vi "AutoEncoder_demo.vi"() -> ()   [LabVIEW 2014]
uses:
  <vilib>/Analysis/baseanly.llb/Vector x A.vi
  <vilib>/Analysis/baseanly.llb/A x Vector.vi
  <vilib>/Analysis/NI_AALBase.lvlib
panel:
  out "XY Graph":cluster{"Array":i32[], dbl[]}(graph)={"Array"=[0, 1, 2, 3, 4, 5, 6, 7, 8, 9, 10, 11, 12, 13, 14, 15, 16, 17, 18, 19, 20, 21, 22, 23, 24, 25, 26, 27, 28, 29, 30, 31, 32, 33, 34, 35, 36, 37, 38, 39, 40, 41, 42, 43, 44, 45, 46, 47, 48, 49, 50, 51, 52, 53, 54, 55, 56, 57, 58, 59, 60, 61, 62, 63, 64, 65, 66, 67, 68, 69, 70, 71, 72, 73, 74, 75, 76, 77, 78, 79, 80, 81, 82, 83, 84, 85, 86, 87, 88, 89, 90, 91, 92, 93, 94, 95, 96, 97, 98, 99, 100, 101, 102, 103, 104, 105, 106, 107, 108, 109, 110, 111, 112, 113, 114, 115, 116, 117, 118, 119, 120, 121, 122, 123, 124, 125, 126, 127, 128, 129, 130, 131, 132, 133, 134, 135, 136, 137, 138, 139, 140, 141, 142, 143, 144, 145, 146, 147, 148, 149, 150], [4.302449553595711, 4.048227484741284, 4.531011299054813, 7.377745697197833, 5.077085434012255, 3.4640879938686306, 2.3579555059462405, 1.6031005412667185, 1.0891350906968578, 0.7396289977203222, 0.5021401051785775, 0.340844705599286, 0.2313319633254815, 0.15699277846584656, 0.10653694142375755, 0.07229445990475002, 0.04905680313771316, 0.03328790003409601, 0.02258753540240982, 0.01532668338521762, 0.010399812316621135, 0.007056697956674369, 0.004788249443257091, 0.003249013786339784, 0.0022045813097912245, 0.0014958933253162794, 0.0010150213329413618, 0.0006887313161076235, 0.0004673310693692157, 0.0003171025081088373, 0.0002151666308504492, 0.00014599917380717274, 9.90663411896271e-05, 6.722055641586043e-05, 4.561191871794354e-05, 3.094958594365995e-05, 2.1000595504256945e-05, 1.4249795896008899e-05, 9.669097646393528e-06, 6.560901500715122e-06, 4.451858575365319e-06, 3.0207826056200174e-06, 2.049735653954206e-06, 1.3908378815287861e-06, 9.43746682957844e-07, 6.403753963009146e-07, 4.3452434133222085e-07, 2.9484505986245243e-07, 2.0006626981382739e-07, 1.357544787687443e-07, 9.211592856751061e-08, 6.250511769704593e-08, 4.241277514149957e-08, 2.8779157426316175e-08, 1.952808890997346e-08, 1.325078707523578e-08, 8.991329075107176e-09, 6.101075692115192e-09, 4.139893199625439e-09, 2.8091322905979654e-09, 1.9061429298950496e-09, 1.2934183593129547e-09, 8.776533856361072e-10, 5.955344848861016e-10, 4.0410240849601025e-10, 2.742056229699723e-10, 1.86063528240424e-10, 1.262547911345823e-10, 8.567078053512786e-11, 5.813246002910622e-11, 3.9445781999185135e-11, 2.676665895782682e-11, 1.8162552403284542e-11, 1.2324148813570466e-11, 8.362283563934942e-12, 5.67446040597241e-12, 3.8502652326963085e-12, 2.6127838590636877e-12, 1.7730125366726473e-12, 1.2031418508383047e-12, 8.164299826220104e-13, 5.538626219870757e-13, 3.758294302867062e-13, 2.550782897881239e-13, 1.7319293256381905e-13, 1.1743050459643337e-13, 7.965906292895184e-14, 5.4198843464053e-14, 3.6641859303897325e-14, 2.5087294302303138e-14, 1.7116730937182402e-14, 1.1708807263476445e-14, 8.099683797877964e-15, 5.511072057502669e-15, 3.751420436264963e-15, 2.6978647938375716e-15, 1.8569289088252427e-15, 1.59250260620481e-15, 1.1240151438116956e-15, 9.914608633805194e-16, 9.773746735086136e-16, 9.662767911105659e-16, 7.570711667007543e-16, 7.570711667007543e-16, 7.570711667007543e-16, 7.570711667007543e-16, 7.570711667007543e-16, 7.570711667007543e-16, 7.570711667007543e-16, 6.888752704931532e-16, 6.888752704931532e-16, 6.888752704931532e-16, 6.888752704931532e-16, 6.888752704931532e-16, 6.888752704931532e-16, 6.888752704931532e-16, 6.888752704931532e-16, 6.888752704931532e-16, 6.888752704931532e-16, 6.888752704931532e-16, 6.888752704931532e-16, 6.888752704931532e-16, 6.888752704931532e-16, 6.888752704931532e-16, 6.521083742145178e-16, 6.521083742145178e-16, 6.521083742145178e-16, 6.521083742145178e-16, 6.521083742145178e-16, 6.521083742145178e-16, 6.521083742145178e-16, 6.521083742145178e-16, 6.521083742145178e-16, 6.521083742145178e-16, 6.521083742145178e-16, 6.521083742145178e-16, 6.521083742145178e-16, 6.521083742145178e-16, 6.521083742145178e-16, 6.521083742145178e-16, 6.521083742145178e-16, 6.521083742145178e-16, 6.521083742145178e-16, 6.521083742145178e-16, 6.521083742145178e-16, 6.521083742145178e-16, 6.521083742145178e-16, 6.521083742145178e-16, 6.521083742145178e-16, 6.521083742145178e-16, 6.521083742145178e-16]}
  out "Waveform Chart":dbl[](graph)=[4.302449553595711, 4.048227484741284, 4.531011299054813, 7.377745697197833, 5.077085434012255, 3.4640879938686306, 2.3579555059462405, 1.6031005412667185, 1.0891350906968578, 0.7396289977203222, 0.5021401051785775, 0.340844705599286, 0.2313319633254815, 0.15699277846584656, 0.10653694142375755, 0.07229445990475002, 0.04905680313771316, 0.03328790003409601, 0.02258753540240982, 0.01532668338521762, 0.010399812316621135, 0.007056697956674369, 0.004788249443257091, 0.003249013786339784, 0.0022045813097912245, 0.0014958933253162794, 0.0010150213329413618, 0.0006887313161076235, 0.0004673310693692157, 0.0003171025081088373, 0.0002151666308504492, 0.00014599917380717274, 9.90663411896271e-05, 6.722055641586043e-05, 4.561191871794354e-05, 3.094958594365995e-05, 2.1000595504256945e-05, 1.4249795896008899e-05, 9.669097646393528e-06, 6.560901500715122e-06, 4.451858575365319e-06, 3.0207826056200174e-06, 2.049735653954206e-06, 1.3908378815287861e-06, 9.43746682957844e-07, 6.403753963009146e-07, 4.3452434133222085e-07, 2.9484505986245243e-07, 2.0006626981382739e-07, 1.357544787687443e-07, 9.211592856751061e-08, 6.250511769704593e-08, 4.241277514149957e-08, 2.8779157426316175e-08, 1.952808890997346e-08, 1.325078707523578e-08, 8.991329075107176e-09, 6.101075692115192e-09, 4.139893199625439e-09, 2.8091322905979654e-09, 1.9061429298950496e-09, 1.2934183593129547e-09, 8.776533856361072e-10, 5.955344848861016e-10, 4.0410240849601025e-10, 2.742056229699723e-10, 1.86063528240424e-10, 1.262547911345823e-10, 8.567078053512786e-11, 5.813246002910622e-11, 3.9445781999185135e-11, 2.676665895782682e-11, 1.8162552403284542e-11, 1.2324148813570466e-11, 8.362283563934942e-12, 5.67446040597241e-12, 3.8502652326963085e-12, 2.6127838590636877e-12, 1.7730125366726473e-12, 1.2031418508383047e-12, 8.164299826220104e-13, 5.538626219870757e-13, 3.758294302867062e-13, 2.550782897881239e-13, 1.7319293256381905e-13, 1.1743050459643337e-13, 7.965906292895184e-14, 5.4198843464053e-14, 3.6641859303897325e-14, 2.5087294302303138e-14, 1.7116730937182402e-14, 1.1708807263476445e-14, 8.099683797877964e-15, 5.511072057502669e-15, 3.751420436264963e-15, 2.6978647938375716e-15, 1.8569289088252427e-15, 1.59250260620481e-15, 1.1240151438116956e-15, 9.914608633805194e-16, 9.773746735086136e-16, 9.662767911105659e-16, 7.570711667007543e-16, 7.570711667007543e-16, 7.570711667007543e-16, 7.570711667007543e-16, 7.570711667007543e-16, 7.570711667007543e-16, 7.570711667007543e-16, 6.888752704931532e-16, 6.888752704931532e-16, 6.888752704931532e-16, 6.888752704931532e-16, 6.888752704931532e-16, 6.888752704931532e-16, 6.888752704931532e-16, 6.888752704931532e-16, 6.888752704931532e-16, 6.888752704931532e-16, 6.888752704931532e-16, 6.888752704931532e-16, 6.888752704931532e-16, 6.888752704931532e-16, 6.888752704931532e-16, 6.521083742145178e-16, 6.521083742145178e-16, 6.521083742145178e-16, 6.521083742145178e-16, 6.521083742145178e-16, 6.521083742145178e-16, 6.521083742145178e-16, 6.521083742145178e-16, 6.521083742145178e-16, 6.521083742145178e-16, 6.521083742145178e-16, 6.521083742145178e-16, 6.521083742145178e-16, 6.521083742145178e-16, 6.521083742145178e-16, 6.521083742145178e-16, 6.521083742145178e-16, 6.521083742145178e-16, 6.521083742145178e-16, 6.521083742145178e-16, 6.521083742145178e-16, 6.521083742145178e-16, 6.521083742145178e-16, 6.521083742145178e-16, 6.521083742145178e-16, 6.521083742145178e-16, 6.521083742145178e-16]
  out "Total Error":dbl[](array[numeric])=[4.302449553595711, 4.048227484741284, 4.531011299054813, 7.377745697197833, 5.077085434012255, 3.4640879938686306, 2.3579555059462405, 1.6031005412667185, 1.0891350906968578, 0.7396289977203222, 0.5021401051785775, 0.340844705599286, 0.2313319633254815, 0.15699277846584656, 0.10653694142375755, 0.07229445990475002, 0.04905680313771316, 0.03328790003409601, 0.02258753540240982, 0.01532668338521762, 0.010399812316621135, 0.007056697956674369, 0.004788249443257091, 0.003249013786339784, 0.0022045813097912245, 0.0014958933253162794, 0.0010150213329413618, 0.0006887313161076235, 0.0004673310693692157, 0.0003171025081088373, 0.0002151666308504492, 0.00014599917380717274, 9.90663411896271e-05, 6.722055641586043e-05, 4.561191871794354e-05, 3.094958594365995e-05, 2.1000595504256945e-05, 1.4249795896008899e-05, 9.669097646393528e-06, 6.560901500715122e-06, 4.451858575365319e-06, 3.0207826056200174e-06, 2.049735653954206e-06, 1.3908378815287861e-06, 9.43746682957844e-07, 6.403753963009146e-07, 4.3452434133222085e-07, 2.9484505986245243e-07, 2.0006626981382739e-07, 1.357544787687443e-07, 9.211592856751061e-08, 6.250511769704593e-08, 4.241277514149957e-08, 2.8779157426316175e-08, 1.952808890997346e-08, 1.325078707523578e-08, 8.991329075107176e-09, 6.101075692115192e-09, 4.139893199625439e-09, 2.8091322905979654e-09, 1.9061429298950496e-09, 1.2934183593129547e-09, 8.776533856361072e-10, 5.955344848861016e-10, 4.0410240849601025e-10, 2.742056229699723e-10, 1.86063528240424e-10, 1.262547911345823e-10, 8.567078053512786e-11, 5.813246002910622e-11, 3.9445781999185135e-11, 2.676665895782682e-11, 1.8162552403284542e-11, 1.2324148813570466e-11, 8.362283563934942e-12, 5.67446040597241e-12, 3.8502652326963085e-12, 2.6127838590636877e-12, 1.7730125366726473e-12, 1.2031418508383047e-12, 8.164299826220104e-13, 5.538626219870757e-13, 3.758294302867062e-13, 2.550782897881239e-13, 1.7319293256381905e-13, 1.1743050459643337e-13, 7.965906292895184e-14, 5.4198843464053e-14, 3.6641859303897325e-14, 2.5087294302303138e-14, 1.7116730937182402e-14, 1.1708807263476445e-14, 8.099683797877964e-15, 5.511072057502669e-15, 3.751420436264963e-15, 2.6978647938375716e-15, 1.8569289088252427e-15, 1.59250260620481e-15, 1.1240151438116956e-15, 9.914608633805194e-16, 9.773746735086136e-16, 9.662767911105659e-16, 7.570711667007543e-16, 7.570711667007543e-16, 7.570711667007543e-16, 7.570711667007543e-16, 7.570711667007543e-16, 7.570711667007543e-16, 7.570711667007543e-16, 6.888752704931532e-16, 6.888752704931532e-16, 6.888752704931532e-16, 6.888752704931532e-16, 6.888752704931532e-16, 6.888752704931532e-16, 6.888752704931532e-16, 6.888752704931532e-16, 6.888752704931532e-16, 6.888752704931532e-16, 6.888752704931532e-16, 6.888752704931532e-16, 6.888752704931532e-16, 6.888752704931532e-16, 6.888752704931532e-16, 6.521083742145178e-16, 6.521083742145178e-16, 6.521083742145178e-16, 6.521083742145178e-16, 6.521083742145178e-16, 6.521083742145178e-16, 6.521083742145178e-16, 6.521083742145178e-16, 6.521083742145178e-16, 6.521083742145178e-16, 6.521083742145178e-16, 6.521083742145178e-16, 6.521083742145178e-16, 6.521083742145178e-16, 6.521083742145178e-16, 6.521083742145178e-16, 6.521083742145178e-16, 6.521083742145178e-16, 6.521083742145178e-16, 6.521083742145178e-16, 6.521083742145178e-16, 6.521083742145178e-16, 6.521083742145178e-16, 6.521083742145178e-16, 6.521083742145178e-16, 6.521083742145178e-16, 6.521083742145178e-16]
  out "by":dbl[](array[numeric])=[0.1520933014698348, -1.3398301547998042, 0.9502810372446283, -1.6761654812494349, 0.06927655170485648, -1.2069484482129365, -0.2101296458734523, 0.21479158877758409] format="%.4f"
  out "Array 2":dbl[][](array[numeric])=[[0.21505248184279538, 1.8505085475091947, 1.5519831697621556, 2.0557146422999626, 1.889129402178558, 2.4061941064539756, 1.9015486562862316, 2.682959459912742], [1.6209332090971538, -2.2962003054879743, 0.6218903541459464, 0.8662162766932792, -0.4996586698333479, -0.7698844002369393, -0.1706204135181342, -1.0625798443384855], [1.1823589897829023, -2.6149253942453607, -2.4858855191228657, -2.4186886279969175, -5.900822976933117, -5.422438514150139, -3.6619219517209465, -3.9138644434139427]] format="%.4f"
  out "Array":dbl[][](array[numeric])=[[0.21505248184279538, 1.4489319414399218, 0.748829957623609, 0.8509848240921414, -1.7250600524449022, -0.80641874210021, -0.9094875861986828, 0.27349982349710206], [1.6209332090971538, -2.2206908717027742, 0.7729092217163482, 1.0927445780488823, 0.1799262342334619, -0.16580892995533109, 0.35794562297827337, -0.6095232416272796], [1.1823589897829023, -1.9209621488513036, -1.0979590283347511, -0.3367988918147455, 0.3448462316134002, 0.12926744900231998, 1.1958207660374547, 0.24991502895040102]] format="%.3f"
  out "Why":dbl[][](array[numeric])=[[0.7503560586047667, 1.2285037642494907, -0.3209409994205742], [1.1234504845287963, -2.062065725977541, 1.7259918231831533], [-0.30049849796394074, -1.3821683505002773, 1.8039756233427267], [0.978245089083142, -1.485443564193626, 0.4480068307926491], [0.8629905310477906, -1.0380734991847376, 0.9660196929785194], [0.6711602207858653, -0.21082311376108656, -1.2147315723991592], [0.20509152550906104, 1.534127050655053, -2.3105573922833047], [1.6494838473290732, -0.02359157177932476, 1.2211020207517798]]
  out "bh":dbl[](array[numeric])=[0.0165027501730751, -1.233081348751569, 1.1995614797139467]
  out "x":dbl[](array[numeric])=[0.0, 0.1111111111111111, 0.2222222222222222, 0.3333333333333333, 1.0, 0.8888888888888888, 0.7777777777777778, 0.6666666666666666]
  out "Wxh":dbl[][](array[numeric])=[[0.21505248184279538, 1.8505085475091947, 1.5519831697621556, 2.0557146422999626, 1.889129402178558, 2.4061941064539756, 1.9015486562862316, 2.682959459912742], [1.6209332090971538, -2.2962003054879743, 0.6218903541459464, 0.8662162766932792, -0.4996586698333479, -0.7698844002369393, -0.1706204135181342, -1.0625798443384855], [1.1823589897829023, -2.6149253942453607, -2.4858855191228657, -2.4186886279969175, -5.900822976933117, -5.422438514150139, -3.6619219517209465, -3.9138644434139427]]
  in  "iterations":i32=150
  in  "rate":dbl=0.011
  out "difference":dbl[][](array[numeric])=[[1.1102230246251565e-16, 0.8888888888888884], [-0.11111111111111133, 0.5555555555555556], [-0.777777777777778, -0.11111111111111083], [-0.44444444444444436, 0.0]] format="%.4f"
  out "output array":dbl[][](array[numeric])=[[-1.1102230246251565e-16, 0.1111111111111116], [0.22222222222222243, 0.33333333333333326], [1.0000000000000002, 0.8888888888888886], [0.7777777777777777, 0.6666666666666666]] format="%.4f"
  out "input array":dbl[][](array[numeric])=[[0.0, 1.0], [0.1111111111111111, 0.8888888888888888], [0.2222222222222222, 0.7777777777777778], [0.3333333333333333, 0.6666666666666666]] format="%0.8f"
  in  "path":path=path "C:/misc/LabVIEW/FILES/TEST/base_sequence_00.txt"
  in  "hidden_units":i32=3
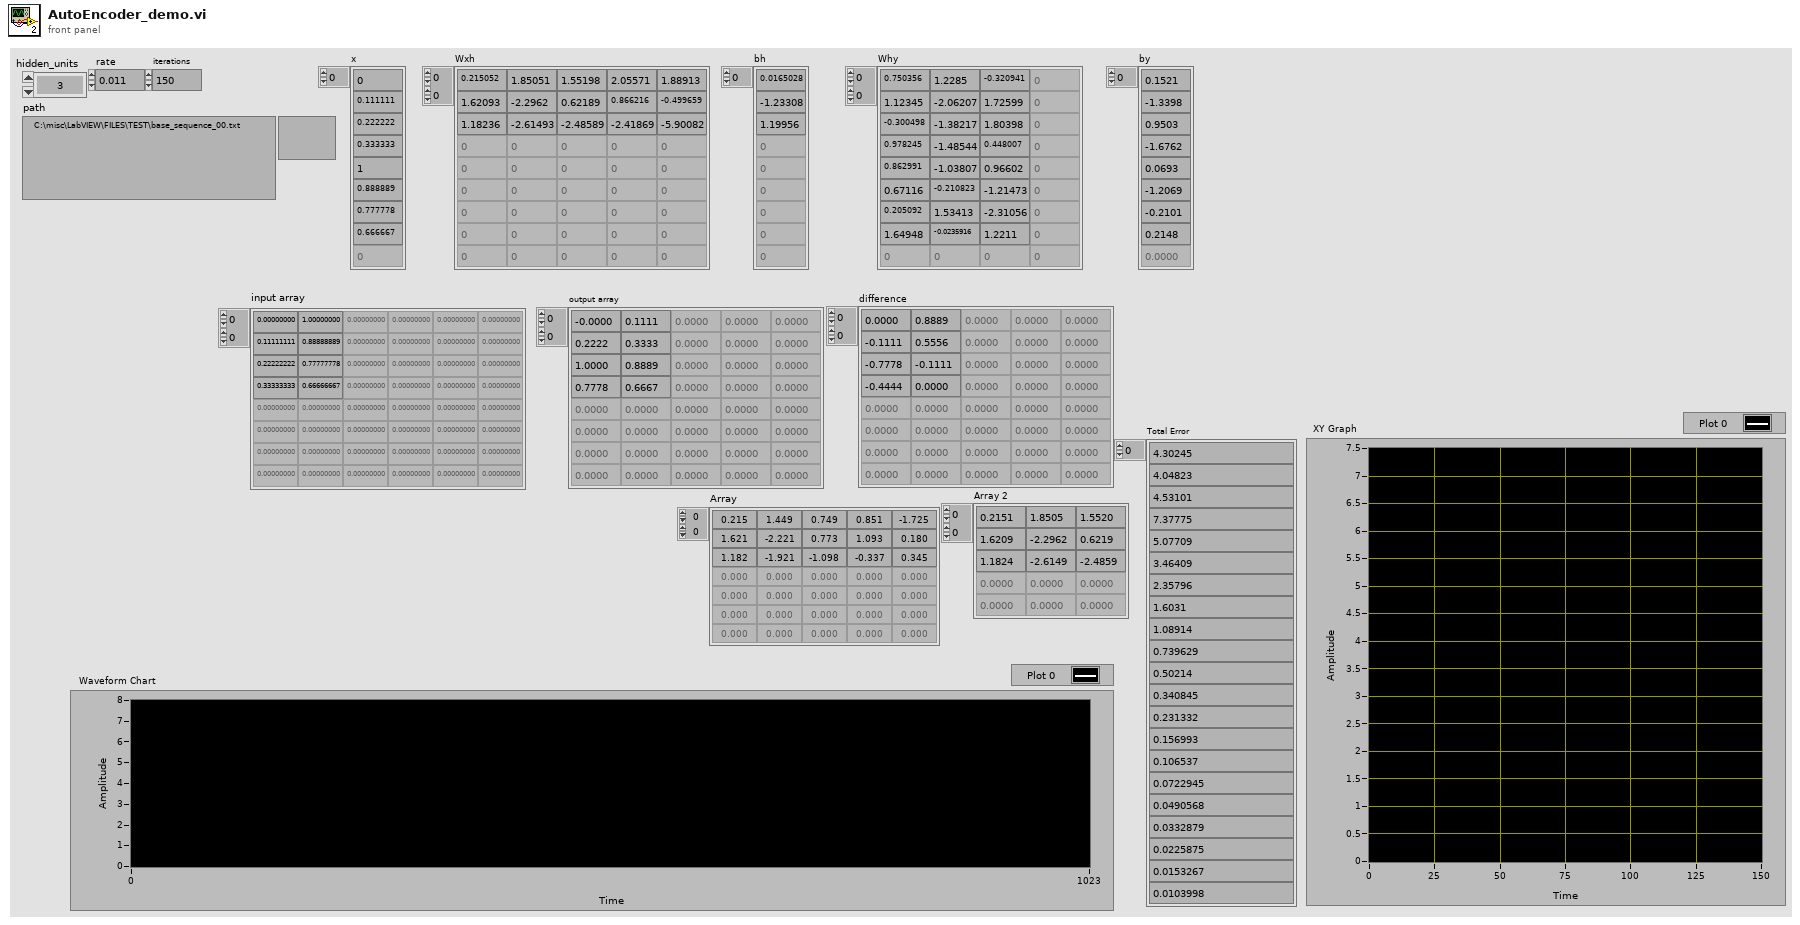
[diagram p1: front panel]
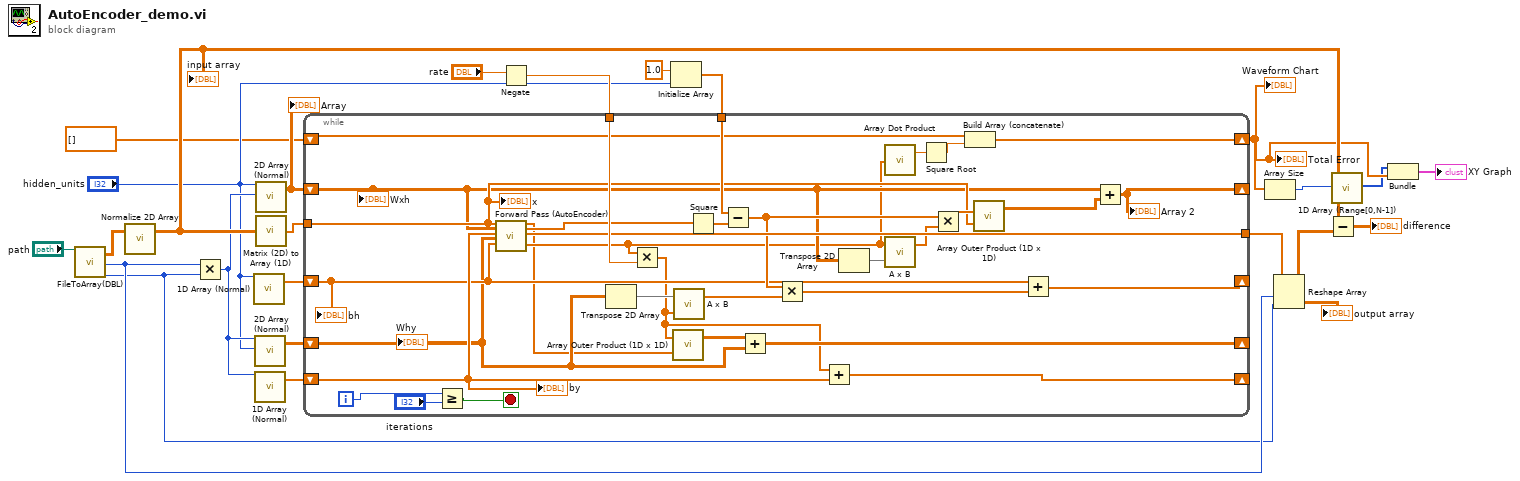
[diagram p0: block diagram]
diagram:
  n1 = call "FileToArray(DBL).vi"("path"="path") -> ("data"=w22:dbl[][], "# rows"=w21:i32, "# cols"=w17:i32)  [unwired: 16 in]
  n2 = call "Normalize 2D Array.vi"("Array"=w22) -> ("Normalized"=w19:dbl[][])  [unwired: 17 in, 1 out]
  "input array" <- w19
  n3 = Multiply(x=w21, y=w17) -> (x*y=w7:i32)
  n4 = call "1D Array (Normal).vi"("samples"="hidden_units") -> ("normal random data"=w24:dbl[])  [unwired: 18 in]
  n5 = call "2D Array (Normal).vi"("rows"=w7, "cols"="hidden_units") -> ("Array"=w9:dbl[][])  [unwired: 17 in]
  n6 = call "1D Array (Normal).vi"("samples"=w7) -> ("normal random data"=w8:dbl[])  [unwired: 18 in]
  n7 = call "2D Array (Normal).vi"("rows"="hidden_units", "cols"=w7) -> ("Array"=w10:dbl[][])  [unwired: 17 in]
  "Array" <- w10
  n8 = call "Matrix (2D) to Array (1D).vi"("Matrix (2D)"=w19) -> ("Array (1D)"=w15:dbl[])  [unwired: 4 in]
  n9 = Negate(x="rate") -> (-x=w13:dbl)
  n10 = Initialize Array(1.0 ("element"), "hidden_units") -> (w11:dbl[])
  n11 = while {
    tunnel: [w36] -> w16
    tunnel: w15 -> [w35]
    shift-right: [w50] -> _
    shift-left: w24 -> [w30]
    tunnel: w13 -> [w57]
    tunnel: w11 -> [w53]
    shift-right: [w44] -> _
    shift-left: w10 -> [w31]
    shift-right: [w46] -> _
    shift-left: w8 -> [w37]
    shift-right: [w45] -> _
    shift-left: w9 -> [w26]
    shift-right: [w41] -> w3
    shift-left: dbl[] [] -> [w40]
    i -> [w48]
    stop <- w49 stop-if-true
    n12 = Greater Or Equal?(x=w48, y="iterations") -> (x >= y?=w49:bool)
    n13 = call "Forward Pass (AutoEncoder).vi"("x"=w35, "Wxh"=w31, "by"=w37, "Wh,xhat"=w26, "bh"=w30) -> ("y"=w25:dbl[], "tanh(y)"=w34:dbl[], "x_hat"=w36:dbl[], "error"=w28:dbl[])  [unwired: 11 in]
    n14 = Transpose 2D Array(2D array=w26) -> (transposed array=w55:dbl[][])
    n15 = Multiply(x=w28, y=w57) -> (x*y=w27:dbl[])
    n16 = call "Array Outer Product (1D x 1D).vi"("array a"=w27, "array b"=w25) -> ("a X b"=w56:dbl[][])  [unwired: 17 in]
    n17 = call-poly <vilib>:"A x B.vi"("Vector"=w27, "A"=w55) -> ("A x Vector"=w52:dbl[])  [unwired: 1 out]
    n18 = Square(x=w34) -> (x^2=w54:dbl[])
    n19 = Subtract(x=w53, y=w54) -> (x-y=w33:dbl[])
    n20 = Add(x=w56, y=w26) -> (x+y=w45:dbl[][])
    n21 = Multiply(x=w33, y=w52) -> (x*y=w29:dbl[])
    n22 = Add(x=w27, y=w37) -> (x+y=w46:dbl[])
    n23 = Transpose 2D Array(2D array=w31) -> (transposed array=w42:dbl[][])
    n24 = call "Array Dot Product.vi"("array a"=w28, "array b"=w28) -> ("a . b"=w39:dbl)  [unwired: 8 in]
    n25 = call-poly <vilib>:"A x B.vi"("Matrix A"=w42, "Vector V'"=w28) -> ("V' x A"=w32:dbl[])  [unwired: 1 out]
    n26 = Square Root(x=w39) -> (sqrt(x)=w38:dbl)
    n27 = Multiply(x=w33, y=w32) -> (x*y=w43:dbl[])
    n28 = Build Array (concatenate)(w40, w38) -> (w41:dbl[])
    n29 = call "Array Outer Product (1D x 1D).vi"("array a"=w43, "array b"=w35) -> ("a X b"=w51:dbl[][])  [unwired: 17 in]
    n30 = Add(x=w30, y=w29) -> (x+y=w50:dbl[])
    n31 = Add(x=w31, y=w51) -> (x+y=w44:dbl[][])
    "Array 2" <- w44
    "Wxh" <- w31
    "x" <- w35
    "bh" <- w30
    "Why" <- w26
    "by" <- w37
  }
  "Total Error" <- w3
  "Waveform Chart" <- w3
  n32 = Array Size(array=w3) -> (size(s)=w4:i32)
  n33 = Reshape Array(w16, w21, w17) -> (w20:dbl[][])
  "output array" <- w20
  n34 = Subtract(x=w19, y=w20) -> (x-y=→"difference":dbl[][])
  n35 = call "1D Array (Range[0,N-1]).vi"("Range"=w4) -> ("Array"=w2:i32[])  [unwired: 18 in]
  n36 = Bundle("Array"=w2, w3) -> (→"XY Graph":cluster{"Array":i32[], dbl[]})  [unwired: 1 in]
